vi "Core.vi"(8 "error in (no error)":errorcluster, 11 "MB in":refnum<class "Master CR.lvclass">) -> (0 "consumer error":errorcluster, 3 "MB out":refnum<class "Master CR.lvclass">)   [LabVIEW 2021, in "Master CR.lvclass"]
uses:
  Master CR.lvclass
  ctl/CR_Core_State.ctl
  Master CR.lvclass/Master CR.ctl
  Status/Run/Write Run.vi
  Status/write/Write write.vi
  Modbus_v121c/Data Model/Device Data Model.lvclass
panel:
  out "MHL error":errorcluster
  in  "write enable":bool=TRUE
  out "CR_Core_State":T1=enum."requests"
  in  "stop":bool
  out "stopped":bool
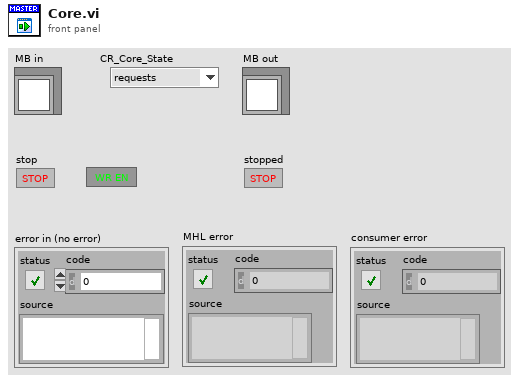
[diagram p1: front panel]
types:
  T1 = typedef "Master CR.lvclass/CR_Core_State.ctl" = enum8{"initialization", "redefine", "standby", "ping", "connect", "wait to reconnect", "wait to reset timeout", "configure", "requests", "close connection", "stop"}
  T2 = typedef "Master CR.lvclass/MB timeouts.ctl" = cluster{"reconn_timeout":i32, "N attempt max":i32, "t_reset_TTL":i32, "period":i32}
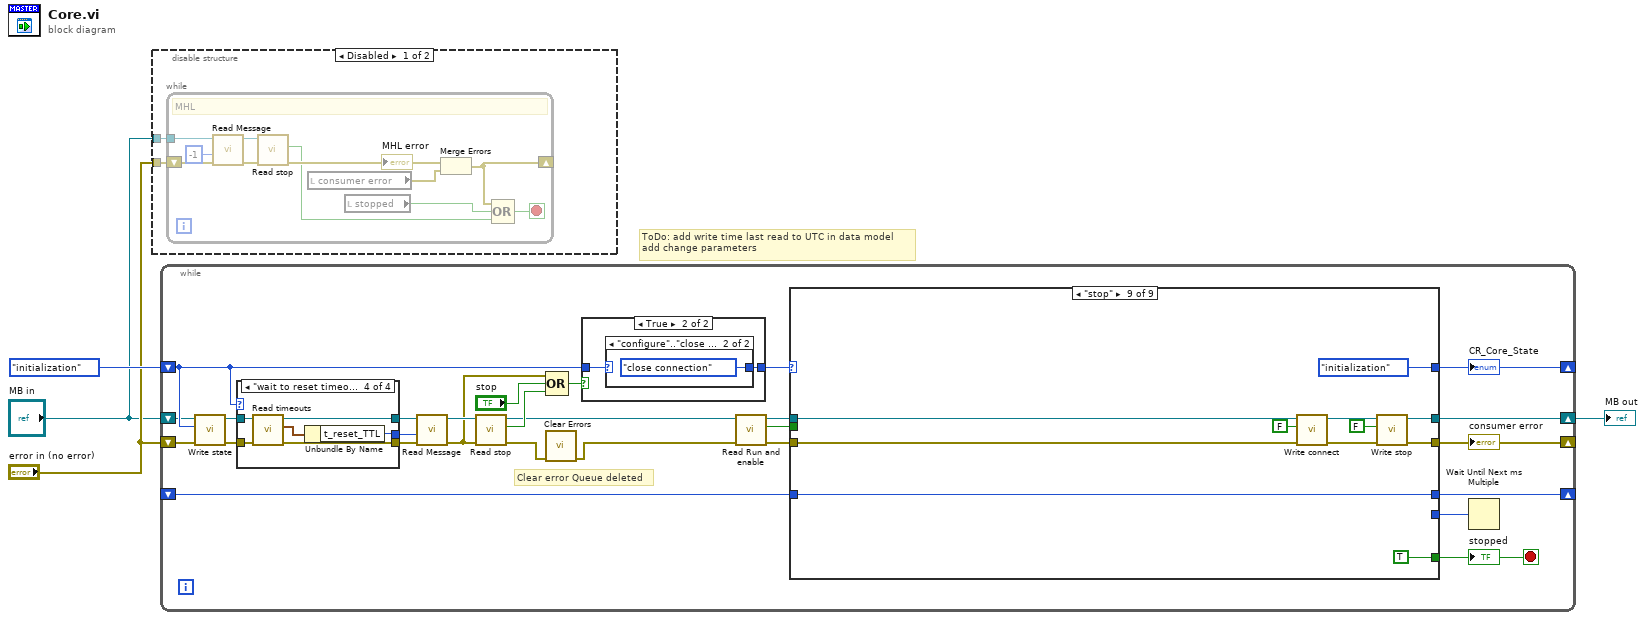
[diagram p0: block diagram]
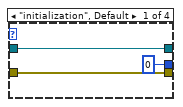
[diagram p3: hidden frame]
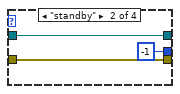
[diagram p4: hidden frame]
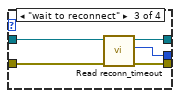
[diagram p5: hidden frame]
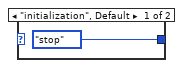
[diagram p7: hidden frame]
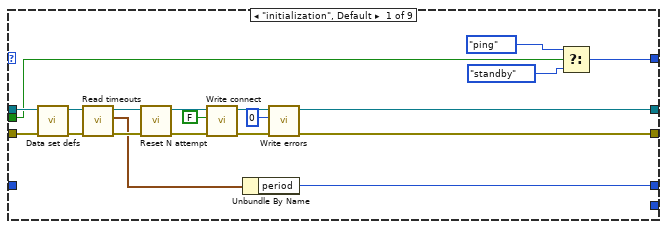
[diagram p8: hidden frame]
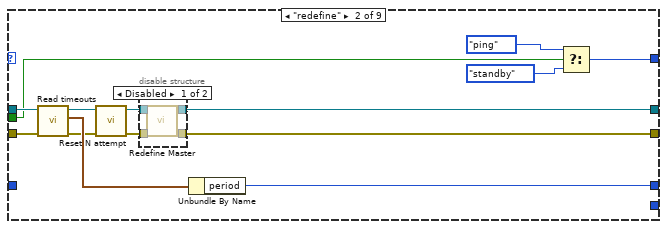
[diagram p9: hidden frame]
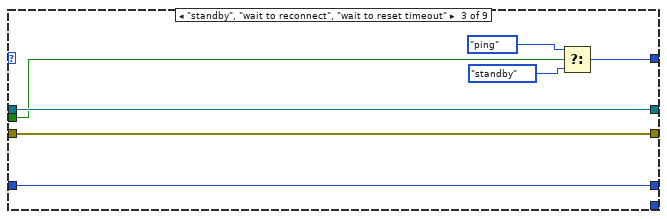
[diagram p11: hidden frame]
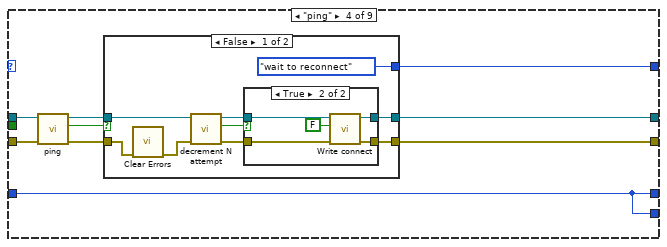
[diagram p12: hidden frame]
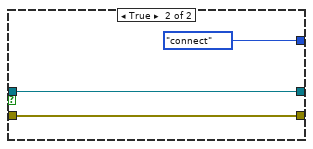
[diagram p14: hidden frame]
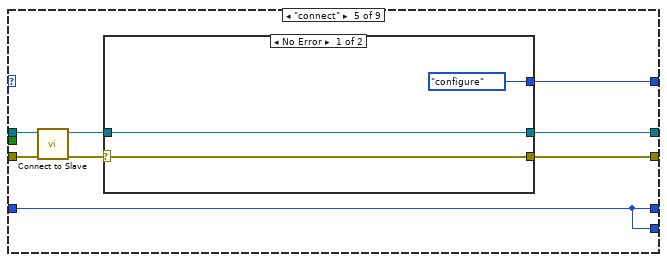
[diagram p15: hidden frame]
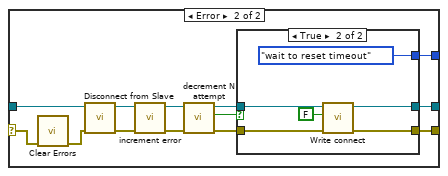
[diagram p16: hidden frame]
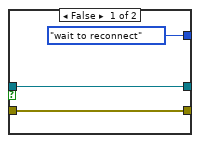
[diagram p17: hidden frame]
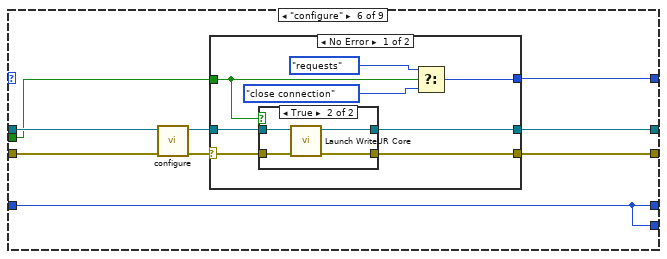
[diagram p18: hidden frame]
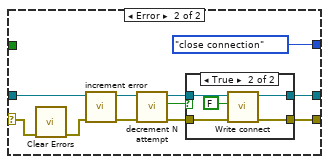
[diagram p20: hidden frame]
diagram:
  # "ToDo: add write time last read to UTC in data model\nadd change parameters"
  n1 = disable-structure shown="Disabled" {
    disable-tunnel: "error in (no error)" -> [w6 _]
    disable-tunnel: "MB in" -> [w5 _]
    frame Disabled {
      n2 = while {
        tunnel: w5 -> [w15]
        shift-right: [w10] -> _
        shift-left: w6 -> [w14]
        stop <- w8 stop-if-true
        # "MHL"
        n3 = call "Read Message.vi"("error in (no error)"=w14, "timeout (0)"=-1, "Master CR in"=w15) -> ("error out"=w13:errorcluster, "Master CR out"=w12:refnum<class "Master CR.lvclass">)  [unwired: 6 in, 1 out]
        n4 = call "Read stop.vi"("error in (no error)"=w13, "Master CR in"=w12) -> ("error out"=w11:errorcluster, "Stop"=w9:bool)  [unwired: 7 in, 1 out]
        "MHL error" <- w11
        n5 = local read "consumer error"() -> (w16:errorcluster)
        n6 = local read "stopped"() -> (w7:bool)
        n7 = Merge Errors(w11, w16) -> (w10:errorcluster)
        n8 = Compound Arithmetic op=OR(w10, w7, w9) -> (w8:bool)
      }
    }
    frame Enabled {
    }
  }
  n9 = while {
    shift-right: [w41] -> w4
    shift-left: "MB in" -> [w19]
    shift-right: [w39] -> _
    shift-left: "error in (no error)" -> [w20]
    shift-right: [w43] -> _
    shift-left: _ -> [w44]
    shift-right: [w40] -> _
    shift-left: CR_Core_State."initialization" ("state") -> [w21]
    stop <- w38 stop-if-true
    # "Clear error Queue deleted"
    n10 = call "Write state.vi"("error in (no error)"=w20, "state"=w21, "Master CR in"=w19) -> ("error out"=w28:errorcluster, "Master CR out"=w27:refnum<class "Master CR.lvclass">)  [unwired: 7 in]
    n11 = case shown="\"wait to reset timeout\"" w21 {
      tunnel: w27 -> [w46 w49 w55 w60]
      tunnel: w28 -> [w45 w48 w54 w59]
      tunnel: [w46 w49 w53 w58] -> w24
      tunnel: [w45 w48 w52 w57] -> w25
      tunnel: [0 ("timeout (0)") -1 ("timeout (0)") w51 w56] -> w26
      frame "initialization", Default {
      }
      frame "standby" {
      }
      frame "wait to reconnect" {
        n12 = call "Read reconn_timeout.vi"("error in (no error)"=w54, "Master CR in"=w55) -> ("error out"=w52:errorcluster, "reconn_timeout"=w51:i32, "Master CR out"=w53:refnum<class "Master CR.lvclass">)  [unwired: 7 in]
      }
      frame "wait to reset timeout" {
        n13 = call "Read timeouts.vi"("error in (no error)"=w59, "Master CR in"=w60) -> ("error out"=w57:errorcluster, "MB timeouts"=w61:T2, "Master CR out"=w58:refnum<class "Master CR.lvclass">)  [unwired: 7 in]
        n14 = Unbundle By Name(w61) -> ("t_reset_TTL"=w56:i32)
      }
    }
    n15 = call "Read Message.vi"("error in (no error)"=w25, "timeout (0)"=w26, "Master CR in"=w24) -> ("error out"=w22:errorcluster, "Master CR out"=w23:refnum<class "Master CR.lvclass">)  [unwired: 6 in, 1 out]
    n16 = call "Read stop.vi"("error in (no error)"=w22, "Master CR in"=w23) -> ("error out"=w30:errorcluster, "Stop"=w33:bool, "Master CR out"=w31:refnum<class "Master CR.lvclass">)  [unwired: 7 in]
    n17 = Compound Arithmetic op=OR(w22, "stop", w33) -> (w32:bool)
    n18 = call <vilib>:"Clear Errors.vi"("error in (no error)"=w30) -> ("error out"=w18:errorcluster)  [unwired: 5 in, 1 out]
    n19 = case shown="True" w32 {
      tunnel: w21 -> [w62 w64]
      tunnel: [w62 w63] -> w29
      frame False {
      }
      frame True {
        n20 = case shown="\"configure\"..\"close connection\"" w64 {
          tunnel: [CR_Core_State."stop" ("MB_TCP_State") CR_Core_State."close connection" ("MB_TCP_State")] -> w63
          frame "initialization", Default {
          }
          frame "configure".."close connection" {
          }
        }
      }
    }
    n21 = call "Read Run and enable.vi"("error in (no error)"=w18, "Master CR in"=w31) -> ("error out"=w37:errorcluster, "Enable and Run"=w35:bool, "Master CR out"=w36:refnum<class "Master CR.lvclass">)  [unwired: 7 in]
    n22 = case shown="\"stop\"" w29 {
      tunnel: [_ _ _ _ _ _ _ _ TRUE] -> w38
      tunnel: w36 -> [w84 w97 w110 w118 w145 w177 w217 w265 w272]
      tunnel: [w69 w89 w110 w122 w149 w183 w224 w257 w275] -> w41
      tunnel: w37 -> [w85 w96 w109 w117 w146 w176 w216 w264 w271]
      tunnel: [w70 w98 w111 w121 w148 w182 w223 w258 CR_Core_State."initialization" ("MB_TCP_State")] -> w40
      tunnel: [w68 w88 w109 w120 w147 w181 w222 w256 w274] -> w39
      tunnel: [w86 w94 w107 w119 w142 w180 w220 w266 w279] -> w43
      tunnel: w44 -> [_ _ w107 w119 w142 w180 w220 w266 w279]
      tunnel: [_ _ _ w119 w142 w180 w220 _ _] -> w42
      tunnel: w35 -> [w67 w87 w108 _ _ w175 w215 w255 _]
      frame "initialization", Default {
        n23 = call "Data set defs.vi"("error in (no error)"=w85, "Master CR in"=w84) -> ("error out"=w79:errorcluster, "Master CR out"=w82:refnum<class "Master CR.lvclass">)  [unwired: 8 in]
        n24 = call "Read timeouts.vi"("error in (no error)"=w79, "Master CR in"=w82) -> ("error out"=w83:errorcluster, "MB timeouts"=w80:T2, "Master CR out"=w81:refnum<class "Master CR.lvclass">)  [unwired: 7 in]
        n25 = call "Reset N attempt.vi"("error in (no error)"=w83, "Master CR in"=w81) -> ("error out"=w77:errorcluster, "Master CR out"=w78:refnum<class "Master CR.lvclass">)  [unwired: 8 in]
        n26 = call "Write connect.vi"("error in (no error)"=w77, "connect"=FALSE, "Master CR in"=w78) -> ("error out"=w75:errorcluster, "Master CR out"=w74:refnum<class "Master CR.lvclass">)  [unwired: 7 in]
        n27 = Unbundle By Name(w80) -> ("period"=w86:i32)
        n28 = call "Write errors.vi"("error in (no error)"=w75, "errors"=0, "Master CR in"=w74) -> ("error out"=w68:errorcluster, "Master CR out"=w69:refnum<class "Master CR.lvclass">)  [unwired: 7 in]
        n29 = Select(t=CR_Core_State."ping" ("MB_TCP_State"), s=w67, f=CR_Core_State."standby" ("MB_TCP_State")) -> (s? t:f=w70:T1)
      }
      frame "redefine" {
        n30 = call "Read timeouts.vi"("error in (no error)"=w96, "Master CR in"=w97) -> ("error out"=w93:errorcluster, "MB timeouts"=w95:T2, "Master CR out"=w92:refnum<class "Master CR.lvclass">)  [unwired: 7 in]
        n31 = call "Reset N attempt.vi"("error in (no error)"=w93, "Master CR in"=w92) -> ("error out"=w90:errorcluster, "Master CR out"=w91:refnum<class "Master CR.lvclass">)  [unwired: 8 in]
        n32 = disable-structure shown="Disabled" {
          disable-tunnel: w91 -> [w104 w106]
          disable-tunnel: w90 -> [w103 w105]
          disable-tunnel: [w102 w106] -> w89
          disable-tunnel: [w101 w105] -> w88
          frame Disabled {
            n33 = call "Redefine Master.vi"("error in (no error)"=w103, "Master CR in"=w104) -> ("error out"=w101:errorcluster, "Master CR out"=w102:refnum<class "Master CR.lvclass">)  [unwired: 8 in]
          }
          frame Enabled {
          }
        }
        n34 = Unbundle By Name(w95) -> ("period"=w94:i32)
        n35 = Select(t=CR_Core_State."ping" ("MB_TCP_State"), s=w87, f=CR_Core_State."standby" ("MB_TCP_State")) -> (s? t:f=w98:T1)
      }
      frame "standby", "wait to reconnect", "wait to reset timeout" {
        n36 = Select(t=CR_Core_State."ping" ("MB_TCP_State"), s=w108, f=CR_Core_State."standby" ("MB_TCP_State")) -> (s? t:f=w111:T1)
      }
      frame "ping" {
        n37 = call-dynamic "ping.vi"("error in (no error)"=w117, "MB_TCP in"=w118) -> ("error out"=w114:errorcluster, "Ping OK"=w115:bool, "MB_TCP out"=w116:refnum<class "Master CR.lvclass">)  [unwired: 7 in]
        n38 = case shown="False" w115 {
          tunnel: w116 -> [w125 w141]
          tunnel: [CR_Core_State."wait to reconnect" ("MB_TCP_State") CR_Core_State."connect" ("MB_TCP_State")] -> w121
          tunnel: [w130 w141] -> w122
          tunnel: [w129 w139] -> w120
          tunnel: w114 -> [w126 w139]
          frame False {
            n39 = call <vilib>:"Clear Errors.vi"("error in (no error)"=w126) -> ("error out"=w124:errorcluster)  [unwired: 5 in, 1 out]
            n40 = call "decrement N attempt.vi"("error in (no error)"=w124, "Master CR in"=w125) -> ("error out"=w127:errorcluster, "=0"=w131:bool, "Master CR out"=w128:refnum<class "Master CR.lvclass">)  [unwired: 7 in]
            n41 = case shown="True" w131 {
              tunnel: w128 -> [w133 w135]
              tunnel: [w133 w138] -> w130
              tunnel: w127 -> [w132 w134]
              tunnel: [w132 w136] -> w129
              frame False {
              }
              frame True {
                n42 = call "Write connect.vi"("error in (no error)"=w134, "connect"=FALSE, "Master CR in"=w135) -> ("error out"=w136:errorcluster, "Master CR out"=w138:refnum<class "Master CR.lvclass">)  [unwired: 7 in]
              }
            }
          }
          frame True {
          }
        }
      }
      frame "connect" {
        n43 = call-dynamic "Connect to Slave.vi"("error in (no error)"=w146, "network master in"=w145) -> ("error out"=w143:errorcluster, "network master out"=w144:refnum<class "Master CR.lvclass">)  [unwired: 8 in]
        n44 = case shown="No Error" w143 {
          selector: w143 -> [w150 w157]
          tunnel: w144 -> [w151 w158]
          tunnel: [CR_Core_State."configure" ("MB_TCP_State") w163] -> w148
          tunnel: [w151 w162] -> w149
          tunnel: [w150 w161] -> w147
          frame No Error {
          }
          frame Error {
            n45 = call <vilib>:"Clear Errors.vi"("error in (no error)"=w157) -> ("error out"=w156:errorcluster)  [unwired: 5 in, 1 out]
            n46 = call-dynamic "Disconnect from Slave.vi"("error in (no error)"=w156, "network master in"=w158) -> ("error out"=w159:errorcluster, "network master out"=w160:refnum<class "Master CR.lvclass">)  [unwired: 8 in]
            n47 = call "increment error.vi"("error in (no error)"=w159, "Master CR in"=w160) -> ("error out"=w155:errorcluster, "Master CR out"=w165:refnum<class "Master CR.lvclass">)  [unwired: 7 in, 1 out]
            n48 = call "decrement N attempt.vi"("error in (no error)"=w155, "Master CR in"=w165) -> ("error out"=w153:errorcluster, "=0"=w164:bool, "Master CR out"=w154:refnum<class "Master CR.lvclass">)  [unwired: 7 in]
            n49 = case shown="True" w164 {
              tunnel: [CR_Core_State."wait to reconnect" ("MB_TCP_State") CR_Core_State."wait to reset timeout" ("MB_TCP_State")] -> w163
              tunnel: w154 -> [w167 w170]
              tunnel: [w167 w173] -> w162
              tunnel: w153 -> [w166 w169]
              tunnel: [w166 w171] -> w161
              frame False {
              }
              frame True {
                n50 = call "Write connect.vi"("error in (no error)"=w169, "connect"=FALSE, "Master CR in"=w170) -> ("error out"=w171:errorcluster, "Master CR out"=w173:refnum<class "Master CR.lvclass">)  [unwired: 7 in]
              }
            }
          }
        }
      }
      frame "configure" {
        n51 = call-dynamic "configure.vi"("error in (no error)"=w176, "Master CR in"=w177) -> ("error out"=w178:errorcluster, "Master CR out"=w179:refnum<class "Master CR.lvclass">)  [unwired: 8 in]
        n52 = case shown="No Error" w178 {
          selector: w178 -> [w186 w206]
          tunnel: [w191 CR_Core_State."close connection" ("MB_TCP_State")] -> w182
          tunnel: [w185 w199] -> w181
          tunnel: w179 -> [w187 w198]
          tunnel: [w184 w200] -> w183
          tunnel: w175 -> [w188 _]
          frame No Error {
            n53 = case shown="True" w188 {
              tunnel: w187 -> [w193 w194]
              tunnel: w186 -> [w192 w196]
              tunnel: [w192 w195] -> w185
              tunnel: [w193 w194] -> w184
              frame False {
              }
              frame True {
                n54 = call "Launch WriteUR Core.vi"("error in"=w196, "Master CR in"=w194) -> ("error out"=w195:errorcluster)  [unwired: 9 in]
              }
            }
            n55 = Select(t=CR_Core_State."requests" ("MB_TCP_State"), s=w188, f=CR_Core_State."close connection" ("MB_TCP_State")) -> (s? t:f=w191:T1)
          }
          frame Error {
            n56 = call <vilib>:"Clear Errors.vi"("error in (no error)"=w206) -> ("error out"=w197:errorcluster)  [unwired: 5 in, 1 out]
            n57 = call "increment error.vi"("error in (no error)"=w197, "Master CR in"=w198) -> ("error out"=w202:errorcluster, "Master CR out"=w201:refnum<class "Master CR.lvclass">)  [unwired: 7 in, 1 out]
            n58 = call "decrement N attempt.vi"("error in (no error)"=w202, "Master CR in"=w201) -> ("error out"=w203:errorcluster, "=0"=w205:bool, "Master CR out"=w204:refnum<class "Master CR.lvclass">)  [unwired: 7 in]
            n59 = case shown="True" w205 {
              tunnel: w204 -> [w209 w214]
              tunnel: [w209 w213] -> w200
              tunnel: w203 -> [w208 w212]
              tunnel: [w208 w210] -> w199
              frame False {
              }
              frame True {
                n60 = call "Write connect.vi"("error in (no error)"=w212, "connect"=FALSE, "Master CR in"=w214) -> ("error out"=w210:errorcluster, "Master CR out"=w213:refnum<class "Master CR.lvclass">)  [unwired: 7 in]
              }
            }
          }
        }
      }
      frame "requests" {
        # "ToDo: add write time last read to UTC in data model"
        n61 = disable-structure shown="Enabled" {
          disable-tunnel: [w225 TRUE] -> _
          frame Disabled {
            n62 = Equal?() -> (x = y?=w225:bool)  [unwired: 2 in]
          }
          frame Enabled {
          }
        }
        n63 = call-dynamic "Requests.vi"("error in (no error)"=w216, "write enable"="write enable", "MB_TCP in"=w217) -> ("error out"=w219:errorcluster, "MB_TCP out"=w221:refnum<class "Master CR.lvclass">)  [unwired: 7 in]
        n64 = case shown="No Error" w219 {
          selector: w219 -> [w232 w247]
          tunnel: [w236 CR_Core_State."close connection" ("MB_TCP_State")] -> w223
          tunnel: w215 -> [w229 _]
          tunnel: [w227 w243] -> w222
          tunnel: w221 -> [w233 w240]
          tunnel: [w230 w244] -> w224
          frame No Error {
            n65 = call "Reset N attempt.vi"("error in (no error)"=w232, "Master CR in"=w233) -> ("error out"=w228:errorcluster, "Master CR out"=w231:refnum<class "Master CR.lvclass">)  [unwired: 8 in]
            n66 = call "Write connect.vi"("error in (no error)"=w228, "connect"=w229, "Master CR in"=w231) -> ("error out"=w227:errorcluster, "Master CR out"=w230:refnum<class "Master CR.lvclass">)  [unwired: 7 in]
            n67 = Select(t=CR_Core_State."requests" ("MB_TCP_State"), s=w229, f=CR_Core_State."close connection" ("MB_TCP_State")) -> (s? t:f=w236:T1)
          }
          frame Error {
            # "clear read error"
            n68 = call <vilib>:"Clear Errors.vi"("error in (no error)"=w247) -> ("error out"=w239:errorcluster)  [unwired: 5 in, 1 out]
            n69 = call "increment error.vi"("error in (no error)"=w239, "Master CR in"=w240) -> ("error out"=w241:errorcluster, "Master CR out"=w246:refnum<class "Master CR.lvclass">)  [unwired: 7 in, 1 out]
            n70 = call "decrement N attempt.vi"("error in (no error)"=w241, "Master CR in"=w246) -> ("error out"=w242:errorcluster, "=0"=w238:bool, "Master CR out"=w245:refnum<class "Master CR.lvclass">)  [unwired: 7 in]
            n71 = case shown="True" w238 {
              tunnel: w245 -> [w249 w254]
              tunnel: [w249 w253] -> w244
              tunnel: w242 -> [w248 w252]
              tunnel: [w248 w250] -> w243
              frame False {
              }
              frame True {
                n72 = call "Write connect.vi"("error in (no error)"=w252, "connect"=FALSE, "Master CR in"=w254) -> ("error out"=w250:errorcluster, "Master CR out"=w253:refnum<class "Master CR.lvclass">)  [unwired: 7 in]
              }
            }
          }
        }
      }
      frame "close connection" {
        n73 = call-dynamic "Disconnect from Slave.vi"("error in (no error)"=w264, "network master in"=w265) -> ("error out"=w256:errorcluster, "network master out"=w257:refnum<class "Master CR.lvclass">)  [unwired: 8 in]
        n74 = disable-structure shown="Enabled" {
          disable-tunnel: [w267 TRUE] -> w259
          frame Disabled {
            n75 = Equal?() -> (x = y?=w267:bool)  [unwired: 2 in]
          }
          frame Enabled {
          }
        }
        n76 = Select(t=CR_Core_State."wait to reconnect" ("MB_TCP_State"), s=w259, f=CR_Core_State."redefine" ("MB_TCP_State")) -> (s? t:f=w261:T1)
        n77 = Select(t=w261, s=w255, f=CR_Core_State."standby" ("MB_TCP_State")) -> (s? t:f=w258:T1)
      }
      frame "stop" {
        n78 = call "Write connect.vi"("error in (no error)"=w271, "connect"=FALSE, "Master CR in"=w272) -> ("error out"=w270:errorcluster, "Master CR out"=w269:refnum<class "Master CR.lvclass">)  [unwired: 7 in]
        n79 = call "Write stop.vi"("error in (no error)"=w270, "Stop"=FALSE, "Master CR in"=w269) -> ("error out"=w274:errorcluster, "Master CR out"=w275:refnum<class "Master CR.lvclass">)  [unwired: 7 in]
      }
    }
    "CR_Core_State" <- w40
    "consumer error" <- w39
    "stopped" <- w38
    n80 = Wait Until Next ms Multiple(millisecond multiple=w42) -> ()  [unwired: 1 out]
  }
  "MB out" <- w4
